vi "数据表比对.vi"(6 "table输入 3":string(combo), 8 "error in (no error)":errorcluster, 9 "查询元素输入":string(combo), 10 "仪器日志参数":string, 11 "table输入":string(combo)) -> (0 "error out":errorcluster, 2 "待发送第一条数据":string[](array[string]), 3 "待发送数据":string[][](table), 4 "获取有效数据":string[][](array[string]))   [LabVIEW 2016]
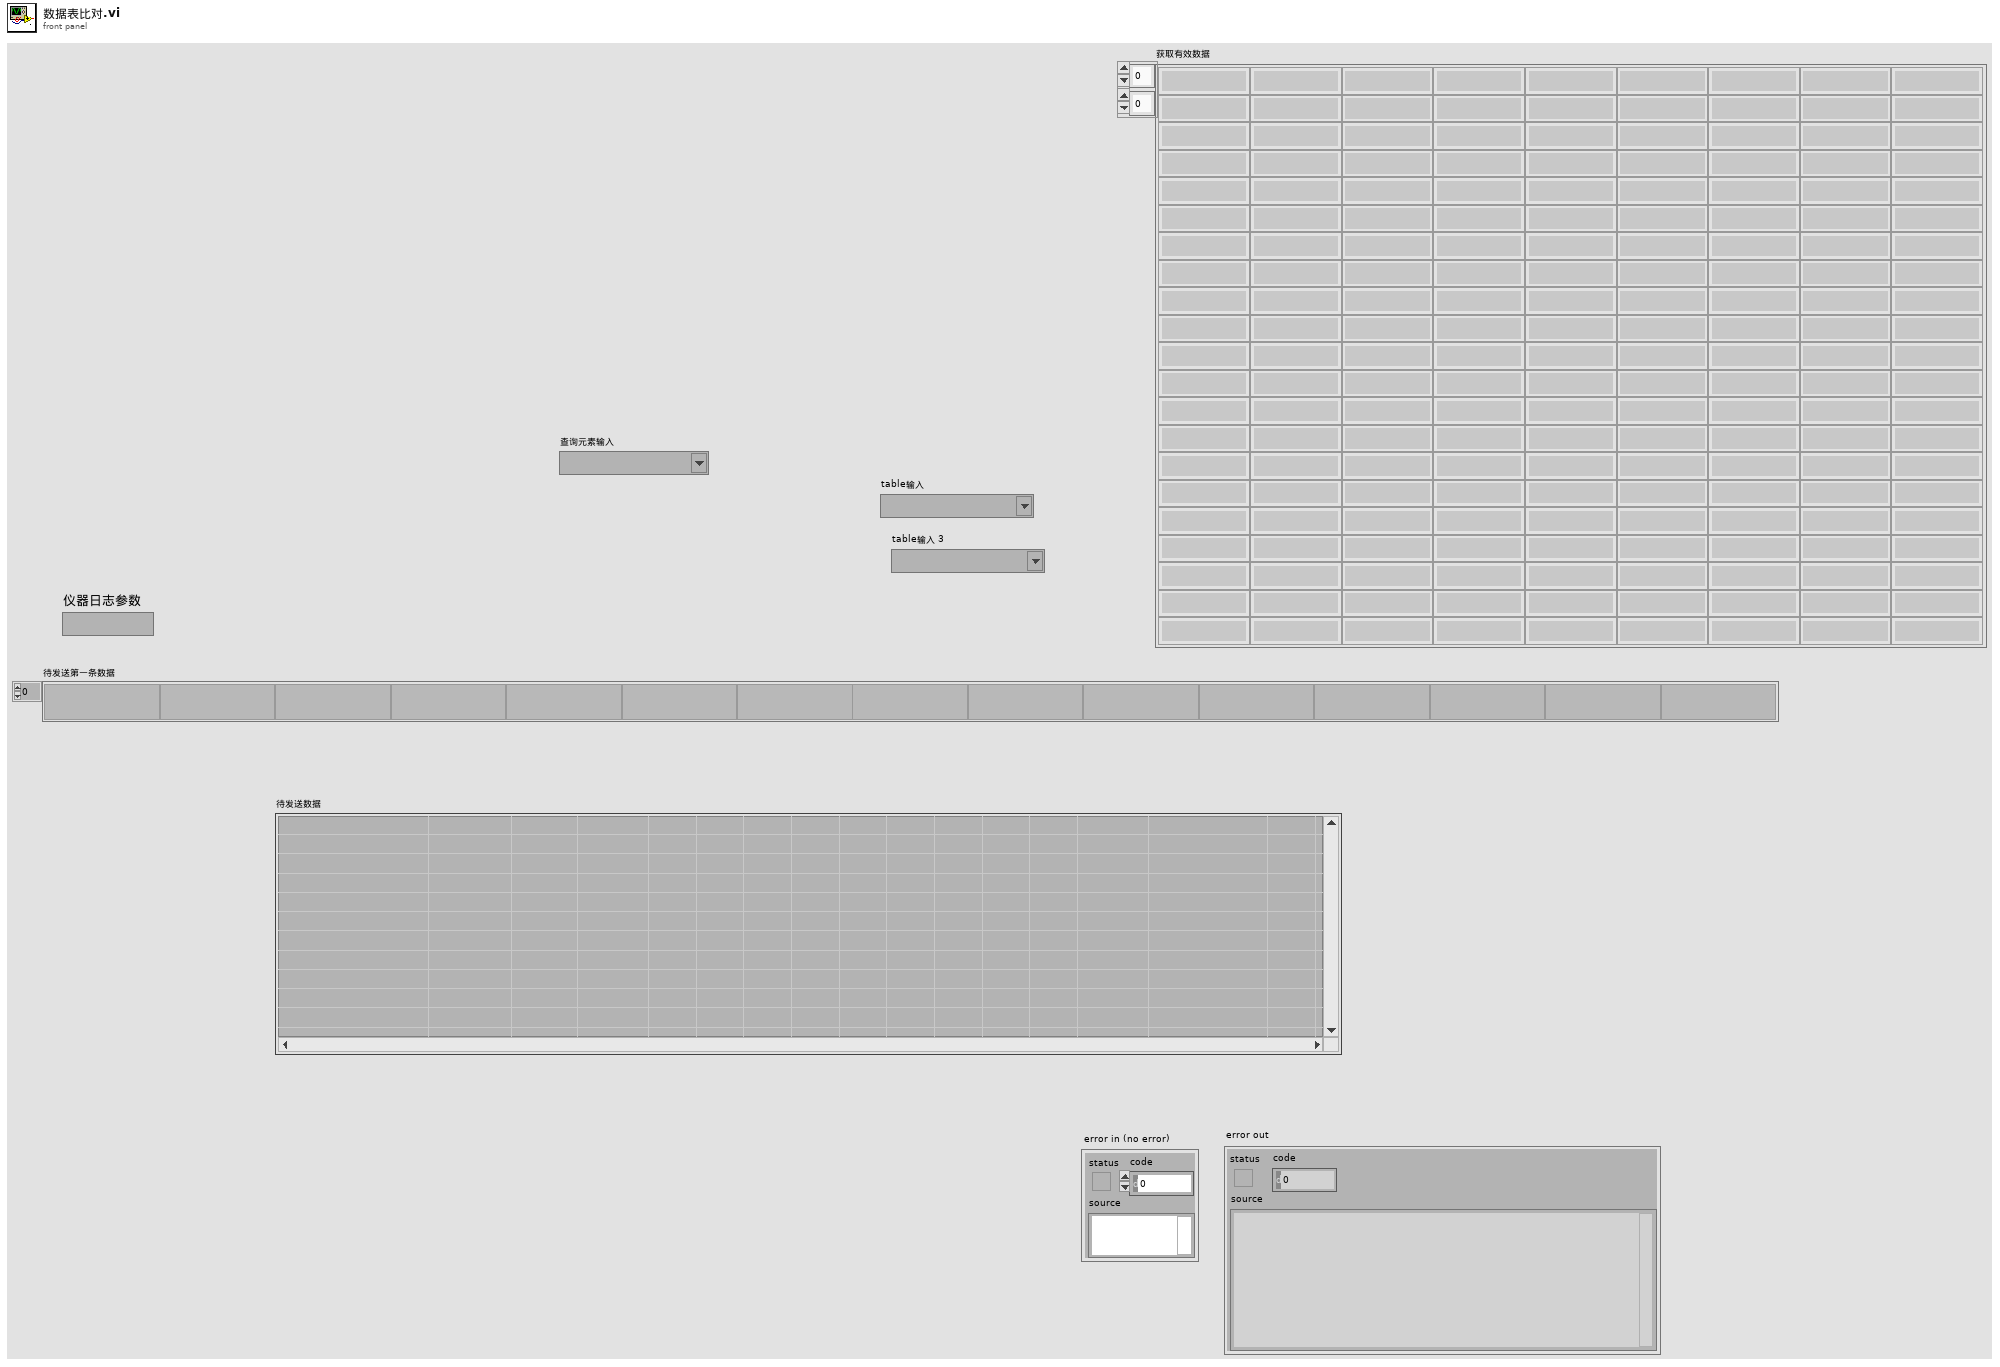
[diagram p1: front panel]
types:
  T1 = typedef "LVDateTimeRec.ctl" = cluster{"秒数的小数部分":dbl, "秒":i32, "分":i32, "时":i32, "日":i32, "月":i32, "年":i32, "天数（周）":i32, "天数（年）":i32, "DST":i32}
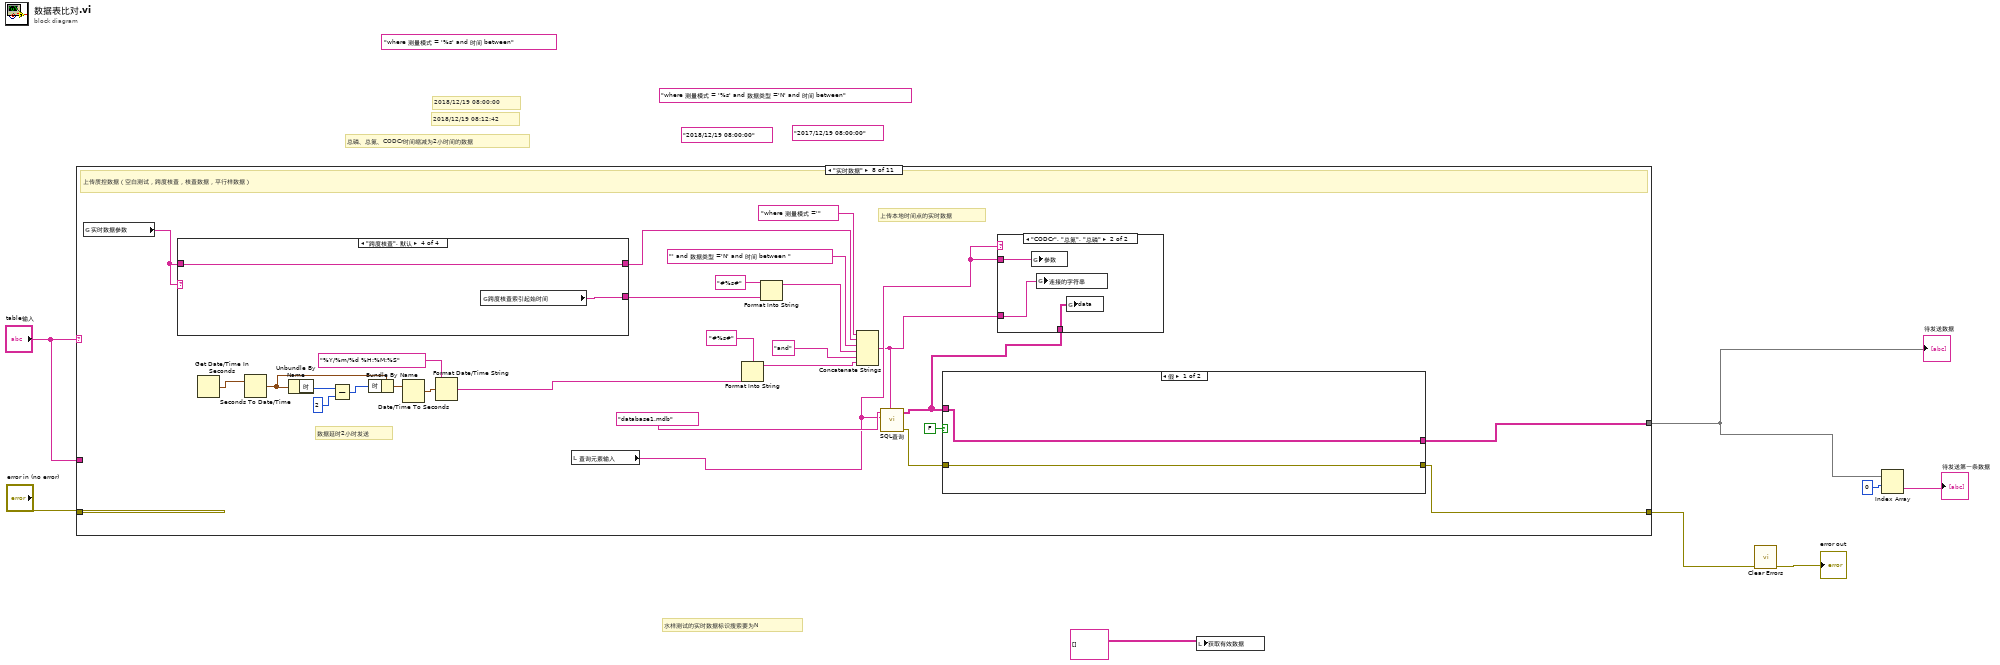
[diagram p0: block diagram]
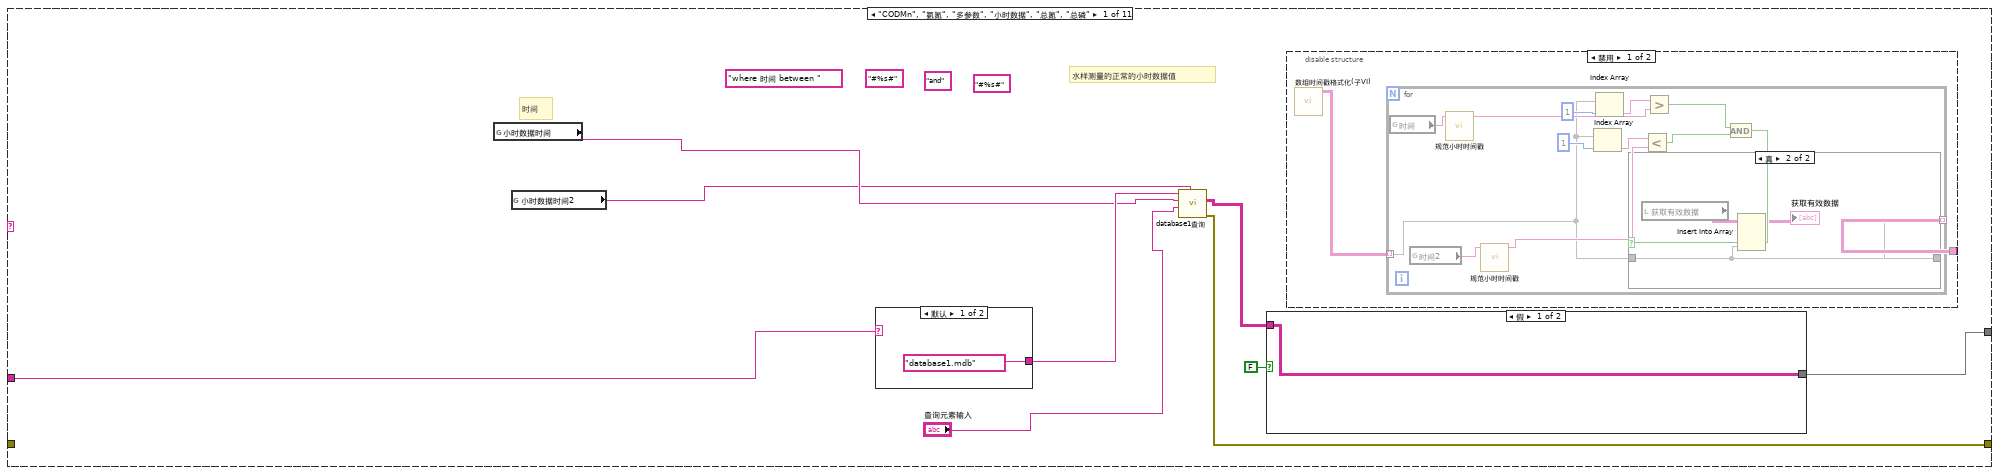
[diagram p2: hidden frame]
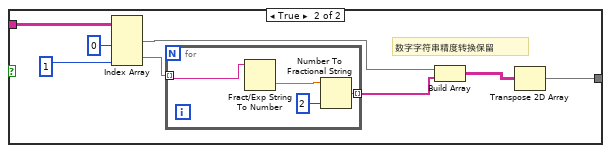
[diagram p3: hidden frame]
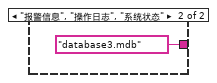
[diagram p6: hidden frame]
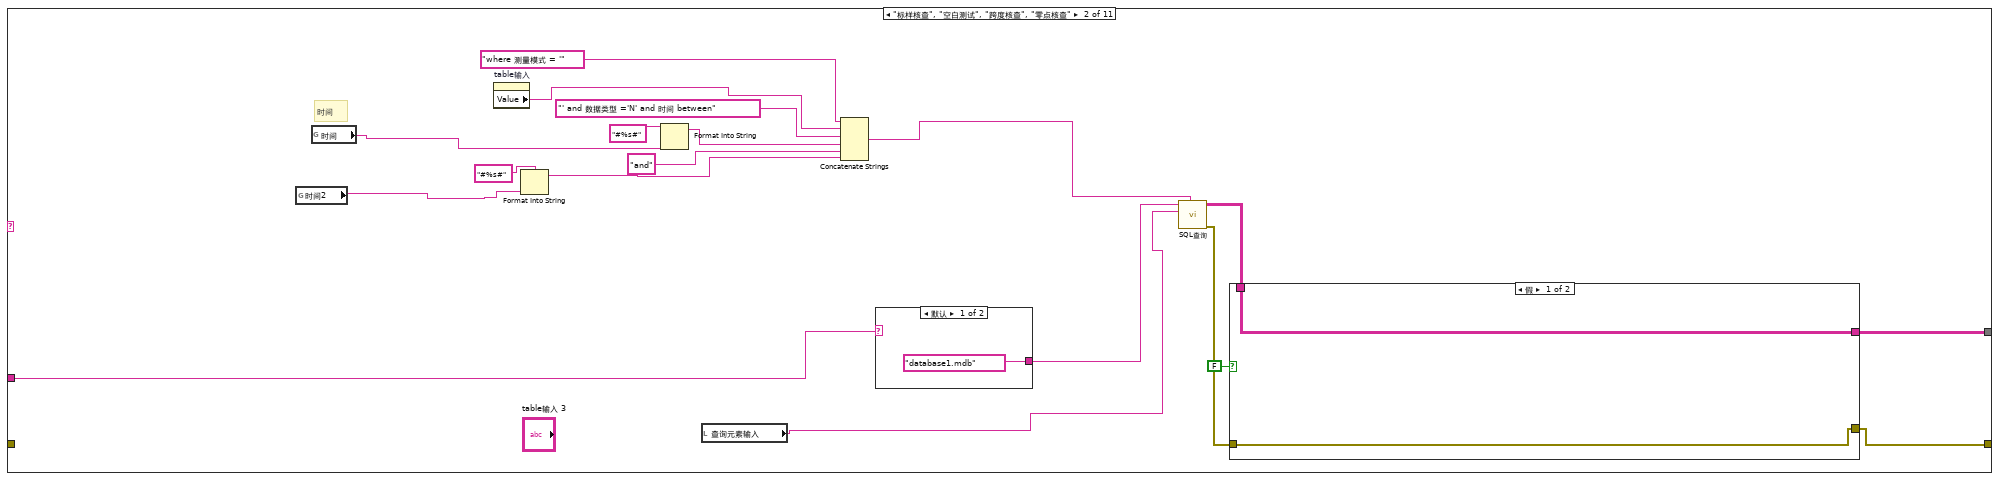
[diagram p7: hidden frame]
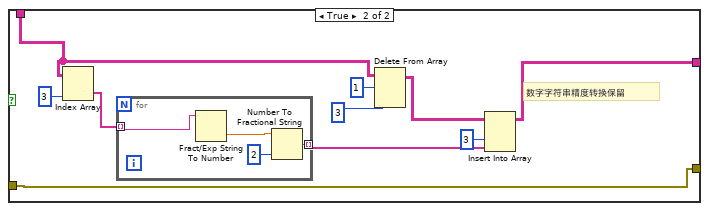
[diagram p8: hidden frame]
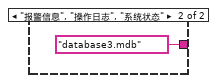
[diagram p9: hidden frame]
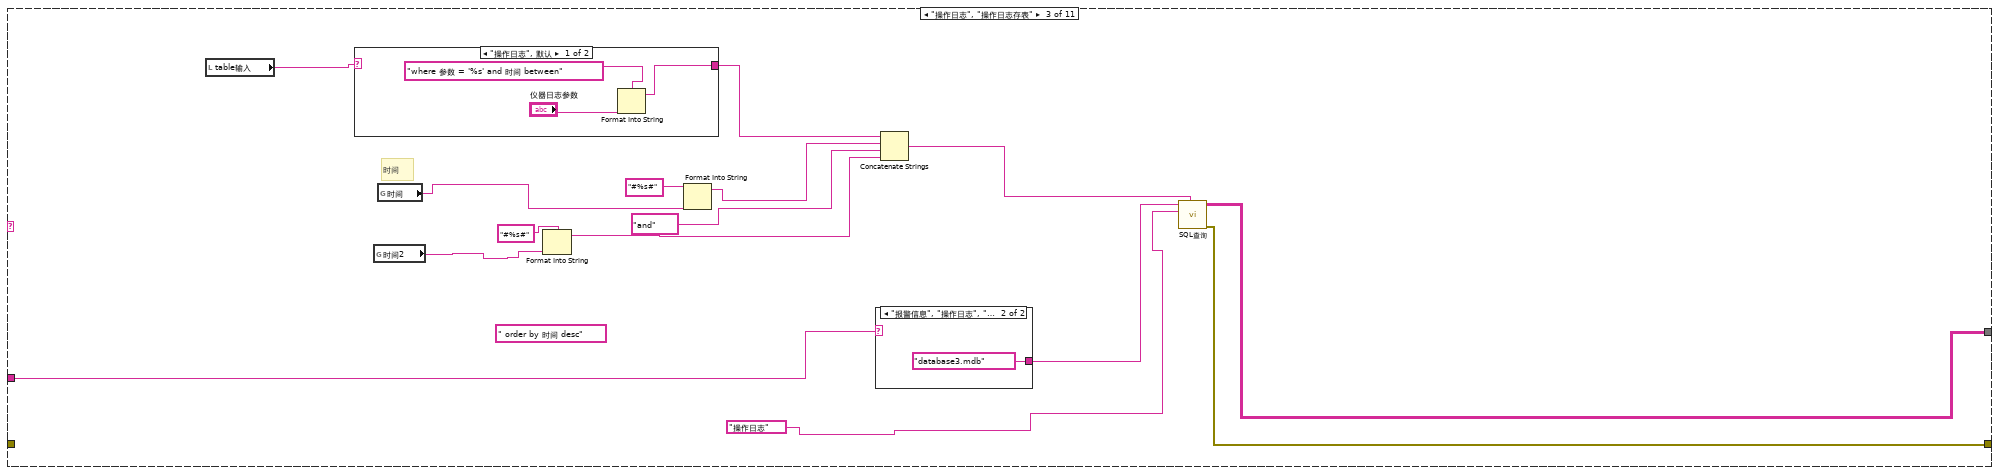
[diagram p10: hidden frame]
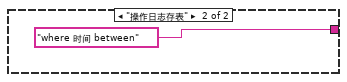
[diagram p11: hidden frame]
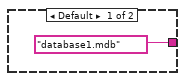
[diagram p12: hidden frame]
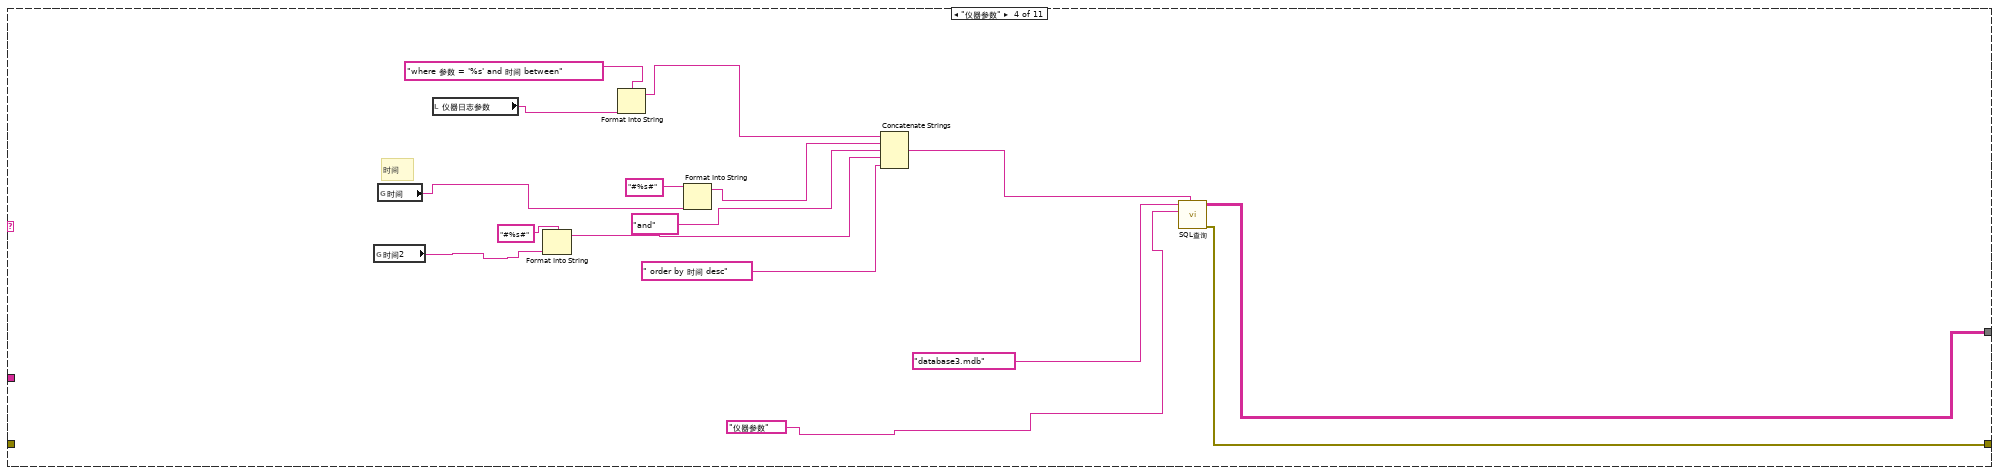
[diagram p13: hidden frame]
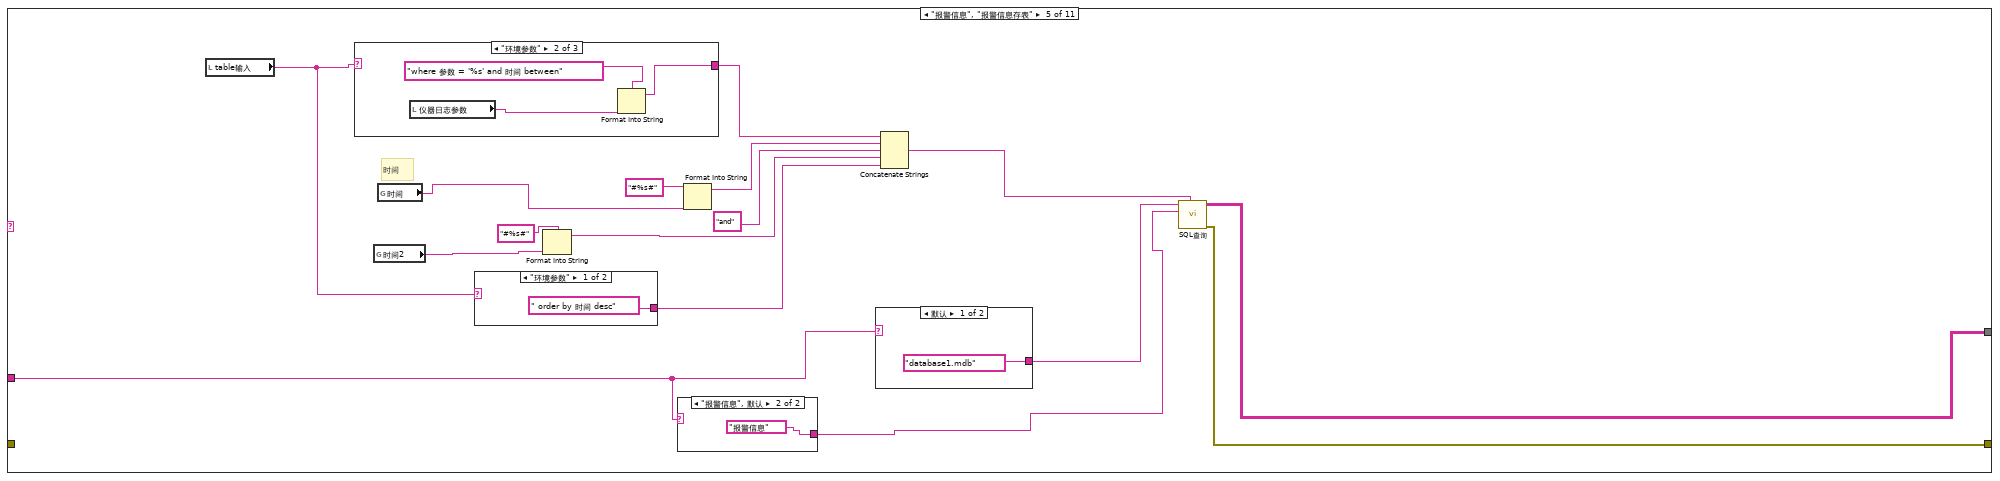
[diagram p14: hidden frame]
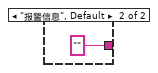
[diagram p15: hidden frame]
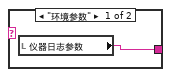
[diagram p16: hidden frame]
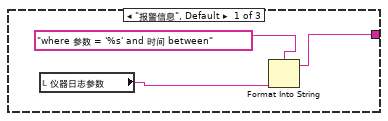
[diagram p17: hidden frame]
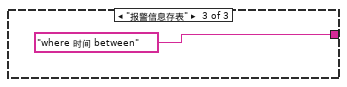
[diagram p18: hidden frame]
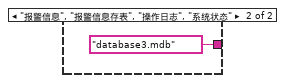
[diagram p19: hidden frame]
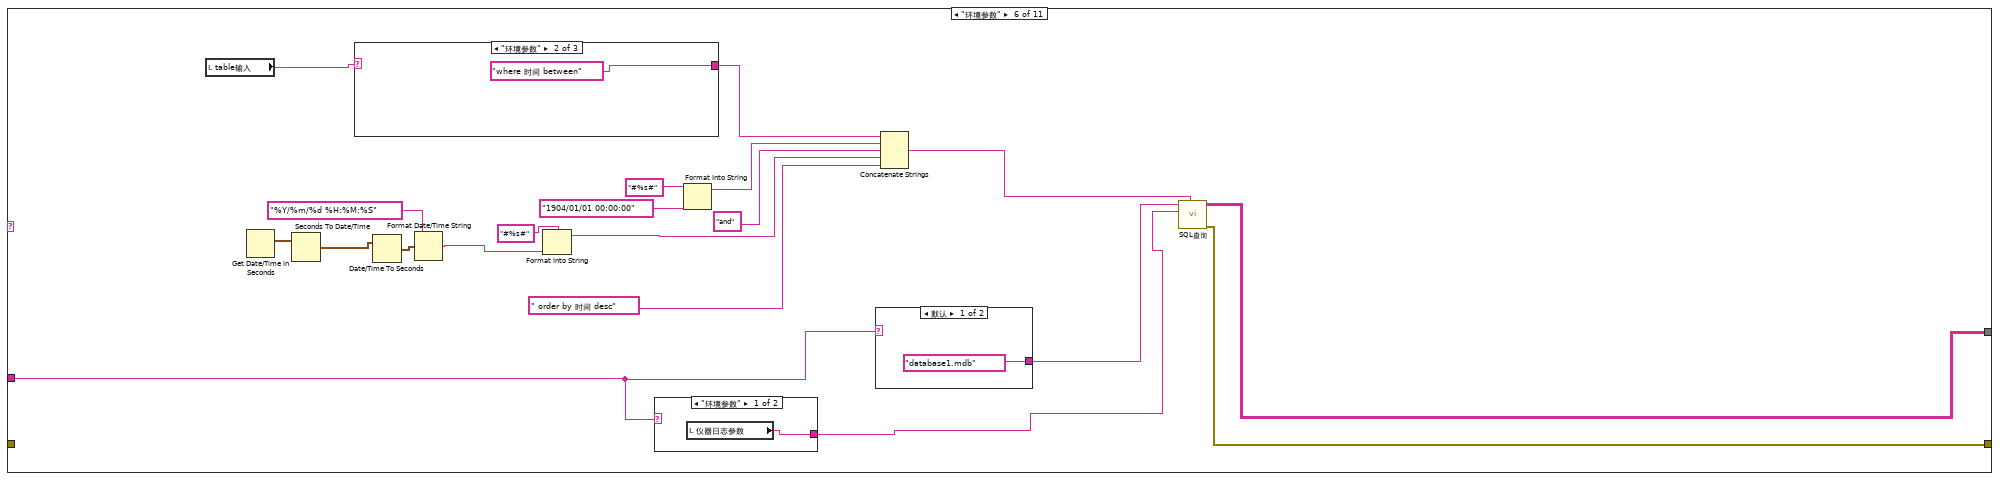
[diagram p20: hidden frame]
diagram:
  (unwired) "where 测量模式 = '%s' and 时间 between" ("condition")
  (unwired) "2017/12/19 08:00:00"
  (unwired) "where 测量模式 = '%s' and 数据类型 ='N' and 时间 between" ("condition")
  (unwired) "2018/12/19 08:00:00"
  # "水样测试的实时数据标识搜索要为N"
  # "2018/12/19 08:00:00"
  # "总磷、总氮、CODCr时间缩减为2小时间的数据"
  # "2018/12/19 08:12:42"
  n1 = case shown="\"实时数据\"" "table输入" {
    tunnel: "error in (no error)" -> [_ _ _ _ _ _ w185 _ _ _ _]
    tunnel: [w14 w55 w100 w123 w139 w172 w185 w201 w266 w309 w349] -> w6
    tunnel: [w10 w58 w98 w121 w137 w170 w183 w204 w269 w312 w351] -> w2
    tunnel: "table输入" -> [w17 w69 w102 _ w127 w162 _ _ _ _ _]
    frame "CODMn", "氨氮", "多参数", "小时数据", "总氮", "总磷" {
      (unwired) "and" ("字符串")
      (unwired) "#%s#" ("初始字符串")
      (unwired) "#%s#" ("初始字符串")
      (unwired) "where 时间 between " ("condition")
      # "水样测量的正常的小时数据值"
      # "时间"
      n2 = global read "全局 水样时间.vi" "小时数据时间"() -> (w13:string)
      n3 = global read "全局 时间2.vi" "小时数据时间2"() -> (w12:string)
      n4 = case shown="默认" w17 {
        tunnel: ["database1.mdb" ("database") "database3.mdb" ("database")] -> w16
        frame Default {
        }
        frame "报警信息", "操作日志", "系统状态" {
        }
      }
      n5 = call "database1查询.vi"("时间2"=w12, "table"="查询元素输入", "时间1"=w13, "database"=w16) -> ("error out"=w14:errorcluster, "data"=w11:string[][])  [unwired: 4 in, 1 out]
      n6 = case shown="假" FALSE {
        tunnel: w11 -> [w18 w26]
        tunnel: [w18 w19] -> w10
        frame False {
        }
        frame True {
          # "数字字符串精度转换保留"
          n7 = Index Array(array=w26, index (col) #1=0 ("禁用的索引 (列)"), index (col) #2=1 ("索引 (列)")) -> (element #1=w22:string[], element #2=w23:string[])  [unwired: 2 in]
          n8 = for {
            tunnel: w23 -> [w28] mode=indexing
            tunnel: [w27] -> w21 mode=indexing
            n9 = Fract/Exp String To Number(string=w28) -> (number=w29:dbl)  [unwired: 3 in, 1 out]
            n10 = Number To Fractional String(number=w29, precision (6)=i16 2 ("精度(6)")) -> (F-format string=w27:string)  [unwired: 2 in]
          }
          n11 = Build Array(w22, w21) -> (w20:string[][])
          n12 = Transpose 2D Array(2D array=w20) -> (transposed array=w19:string[][])
        }
      }
      n13 = disable-structure shown="禁用" {
        disable-tunnel: [w31 _] -> _
        frame Disabled {
          n14 = call "数组时间戳格式化(子VI).vi"() -> ("待发送数据输出"=w32:string[][])  [unwired: 11 in]
          n15 = for {
            tunnel: w32 -> [w33] mode=indexing
            tunnel: [w35] -> w31 mode=indexing
            n16 = global read "全局 水样时间.vi" "时间"() -> (w39:string)
            n17 = global read "全局 时间2.vi" "时间2"() -> (w37:string)
            n18 = call "规范小时时间戳.vi"("字符串"=w39) -> ("result string"=w38:string)  [unwired: 10 in]
            n19 = call "规范小时时间戳.vi"("字符串"=w37) -> ("result string"=w36:string)  [unwired: 10 in]
            n20 = Index Array(array=w33, index=1 ("索引")) -> (element=w42:string)
            n21 = Index Array(array=w33, index=1 ("索引")) -> (element=w44:string)
            n22 = Less?(x=w42, y=w36) -> (x < y?=w41:bool)
            n23 = Greater?(x=w44, y=w38) -> (0:w40:bool)
            n24 = And(x=w40, y=w41) -> (x .and. y?=w34:bool)
            n25 = case shown="真" w34 {
              tunnel: w33 -> [_ w48]
              tunnel: [_ w48] -> w35
              frame False {
              }
              frame True {
                n26 = local read "获取有效数据"() -> (w47:string[][])
                n27 = Insert Into Array(array=w47, new element=w48) -> (→"获取有效数据":string[][])  [unwired: 2 in]
              }
            }
          }
        }
        frame Enabled {
        }
      }
    }
    frame "标样核查", "空白测试", "跨度核查", "零点核查" {
      # "时间"
      n28 = global read "全局 时间2.vi" "时间2"() -> (w60:string)
      n29 = global read "全局 水样时间.vi" "时间"() -> (w61:string)
      n30 = property on="table输入" class="CmbBox"() -> ("Value"=w51:string)  [unwired: 2 in, 2 out]
      n31 = Format Into String(format string="#%s#" ("初始字符串"), w60) -> (resulting string=w63:string)  [unwired: 2 in, 1 out]
      n32 = Format Into String(format string="#%s#" ("初始字符串"), w61) -> (resulting string=w67:string)  [unwired: 2 in, 1 out]
      n33 = local read "查询元素输入"() -> (w54:string)
      n34 = Concatenate Strings("where 测量模式 = '" ("condition"), w51, "' and 数据类型 ='N' and 时间 between" ("字符串"), w67, "and" ("字符串"), w63) -> (w62:string)
      n35 = case shown="默认" w69 {
        tunnel: ["database1.mdb" ("database") "database3.mdb" ("database")] -> w68
        frame Default {
        }
        frame "报警信息", "操作日志", "系统状态" {
        }
      }
      n36 = call "SQL查询.vi"("condition"=w62, "table输入"=w54, "database"=w68) -> ("error out"=w56:errorcluster, "data"=w59:string[][])  [unwired: 7 in]
      n37 = case shown="假" FALSE {
        tunnel: w59 -> [w71 w74]
        tunnel: [w71 w73] -> w58
        tunnel: [w70 w72] -> w55
        tunnel: w56 -> [w70 w72]
        frame False {
        }
        frame True {
          # "数字字符串精度转换保留"
          n38 = Index Array(array=w74, index (col)=3 ("禁用的索引 (列)")) -> (element=w80:string[])  [unwired: 1 in]
          n39 = for {
            tunnel: w80 -> [w83] mode=indexing
            tunnel: [w82] -> w76 mode=indexing
            n40 = Fract/Exp String To Number(string=w83) -> (number=w84:dbl)  [unwired: 3 in, 1 out]
            n41 = Number To Fractional String(number=w84, precision (6)=i16 2 ("精度(6)")) -> (F-format string=w82:string)  [unwired: 2 in]
          }
          n42 = Delete From Array(array=w74, length=1 ("长度"), index (col)=3 ("禁用的索引 (列)")) -> (array with subset deleted=w77:string[][])  [unwired: 1 in, 1 out]
          n43 = Insert Into Array(array=w77, index (col)=3 ("禁用的索引 (列)"), new element=w76) -> (w73:string[][])  [unwired: 1 in]
        }
      }
    }
    frame "操作日志", "操作日志存表" {
      (unwired) " order by 时间 desc" ("字符串")
      # "时间"
      n44 = local read "table输入"() -> (w90:string)
      n45 = case shown="\"操作日志\", 默认" w90 {
        tunnel: [w103 "where 时间 between" ("condition")] -> w89
        frame "操作日志", Default {
          n46 = Format Into String(format string="where 参数 = '%s' and 时间 between" ("condition"), "仪器日志参数") -> (resulting string=w103:string)  [unwired: 2 in, 1 out]
        }
        frame "操作日志存表" {
        }
      }
      n47 = global read "全局 时间2.vi" "时间2"() -> (w91:string)
      n48 = global read "全局 水样时间.vi" "时间"() -> (w92:string)
      n49 = Format Into String(format string="#%s#" ("初始字符串"), w91) -> (resulting string=w93:string)  [unwired: 2 in, 1 out]
      n50 = Format Into String(format string="#%s#" ("初始字符串"), w92) -> (resulting string=w97:string)  [unwired: 2 in, 1 out]
      n51 = case shown="\"报警信息\", \"操作日志\", \"操作日志存表\", \"系统状态\"" w102 {
        tunnel: ["database1.mdb" ("database") "database3.mdb" ("database")] -> w101
        frame Default {
        }
        frame "报警信息", "操作日志", "操作日志存表", "系统状态" {
        }
      }
      n52 = Concatenate Strings(w89, w97, "and" ("字符串"), w93) -> (w99:string)
      n53 = call "SQL查询.vi"("condition"=w99, "table输入"="操作日志", "database"=w101) -> ("error out"=w100:errorcluster, "data"=w98:string[][])  [unwired: 7 in]
    }
    frame "仪器参数" {
      # "时间"
      n54 = global read "全局 时间2.vi" "时间2"() -> (w114:string)
      n55 = global read "全局 水样时间.vi" "时间"() -> (w115:string)
      n56 = local read "仪器日志参数"() -> (w109:string)
      n57 = Format Into String(format string="#%s#" ("初始字符串"), w114) -> (resulting string=w116:string)  [unwired: 2 in, 1 out]
      n58 = Format Into String(format string="where 参数 = '%s' and 时间 between" ("condition"), w109) -> (resulting string=w113:string)  [unwired: 2 in, 1 out]
      n59 = Format Into String(format string="#%s#" ("初始字符串"), w115) -> (resulting string=w120:string)  [unwired: 2 in, 1 out]
      n60 = Concatenate Strings(w113, w120, "and" ("字符串"), w116, " order by 时间 desc" ("字符串")) -> (w122:string)
      n61 = call "SQL查询.vi"("condition"=w122, "table输入"="仪器参数", "database"="database3.mdb") -> ("error out"=w123:errorcluster, "data"=w121:string[][])  [unwired: 7 in]
    }
    frame "报警信息", "报警信息存表" {
      # "时间"
      n62 = local read "table输入"() -> (w126:string)
      n63 = case shown="\"环境参数\"" w126 {
        tunnel: [w146 w149 "where 时间 between" ("condition")] -> w129
        frame "报警信息", Default {
          n64 = local read "仪器日志参数"() -> (w145:string)
          n65 = Format Into String(format string="where 参数 = '%s' and 时间 between" ("condition"), w145) -> (resulting string=w146:string)  [unwired: 2 in, 1 out]
        }
        frame "环境参数" {
          n66 = local read "仪器日志参数"() -> (w148:string)
          n67 = Format Into String(format string="where 参数 = '%s' and 时间 between" ("condition"), w148) -> (resulting string=w149:string)  [unwired: 2 in, 1 out]
        }
        frame "报警信息存表" {
        }
      }
      n68 = global read "全局 时间2.vi" "时间2"() -> (w130:string)
      n69 = global read "全局 水样时间.vi" "时间"() -> (w131:string)
      n70 = case shown="\"环境参数\"" w126 {
        tunnel: [" order by 时间 desc" ("字符串") "" ("仪器日志参数")] -> w125
        frame "环境参数" {
        }
        frame "报警信息", Default {
        }
      }
      n71 = Format Into String(format string="#%s#" ("初始字符串"), w130) -> (resulting string=w132:string)  [unwired: 2 in, 1 out]
      n72 = case shown="\"报警信息\", 默认" w127 {
        tunnel: [w143 "报警信息" ("table输入")] -> w128
        frame "环境参数" {
          n73 = local read "仪器日志参数"() -> (w143:string)
        }
        frame "报警信息", Default {
        }
      }
      n74 = Format Into String(format string="#%s#" ("初始字符串"), w131) -> (resulting string=w136:string)  [unwired: 2 in, 1 out]
      n75 = case shown="默认" w127 {
        tunnel: ["database1.mdb" ("database") "database3.mdb" ("database")] -> w140
        frame Default {
        }
        frame "报警信息", "报警信息存表", "操作日志", "系统状态" {
        }
      }
      n76 = Concatenate Strings(w129, w136, "and" ("字符串"), w132, w125) -> (w138:string)
      n77 = call "SQL查询.vi"("condition"=w138, "table输入"=w128, "database"=w140) -> ("error out"=w139:errorcluster, "data"=w137:string[][])  [unwired: 7 in]
    }
    frame "环境参数" {
      n78 = local read "table输入"() -> (w161:string)
      n79 = Get Date/Time In Seconds() -> (seconds since 1Jan1904=w158:timestamp)
      n80 = Seconds To Date/Time(time stamp (now)=w158) -> (date time rec=w155:T1)  [unwired: 1 in]
      n81 = case shown="\"环境参数\"" w161 {
        tunnel: [w177 "where 时间 between" ("condition") "where 时间 between" ("condition")] -> w164
        frame "报警信息", Default {
          n82 = local read "仪器日志参数"() -> (w176:string)
          n83 = Format Into String(format string="where 参数 = '%s' and 时间 between" ("condition"), w176) -> (resulting string=w177:string)  [unwired: 2 in, 1 out]
        }
        frame "环境参数" {
        }
        frame "报警信息存表" {
        }
      }
      n84 = Date/Time To Seconds(2:w155) -> (0:w157:timestamp)  [unwired: 1 in]
      n85 = Format Date/Time String(time format string (%c)="%Y/%m/%d %H:%M:%S" ("时间格式字符串(%c)"), seconds (now)=w157) -> (date/time string=w154:string)  [unwired: 1 in]
      n86 = Format Into String(format string="#%s#" ("初始字符串"), w154) -> (resulting string=w165:string)  [unwired: 2 in, 1 out]
      n87 = case shown="\"环境参数\"" w162 {
        tunnel: [w174 "报警信息" ("table输入")] -> w163
        frame "环境参数" {
          n88 = local read "仪器日志参数"() -> (w174:string)
        }
        frame "报警信息", Default {
        }
      }
      n89 = Format Into String(format string="#%s#" ("初始字符串"), "1904/01/01 00:00:00") -> (resulting string=w169:string)  [unwired: 2 in, 1 out]
      n90 = case shown="默认" w162 {
        tunnel: ["database1.mdb" ("database") "database3.mdb" ("database")] -> w173
        frame Default {
        }
        frame "报警信息", "报警信息存表", "操作日志", "系统状态" {
        }
      }
      n91 = Concatenate Strings(w164, w169, "and" ("字符串"), w165, " order by 时间 desc" ("字符串")) -> (w171:string)
      n92 = call "SQL查询.vi"("condition"=w171, "table输入"=w163, "database"=w173) -> ("error out"=w172:errorcluster, "data"=w170:string[][])  [unwired: 7 in]
    }
    frame Default {
      # "时间格式转换"
      n93 = local read "待发送数据"() -> (w184:string[][])
      n94 = call "数组时间戳格式化(子VI).vi"("待发送数据输入"=w184) -> ("待发送数据输出"=w183:string[][])  [unwired: 10 in]
    }
    frame "实时数据" {
      # "数据延时2小时发送"
      # "上传本地时间点的实时数据"
      # "上传质控数据（空白测试，跨度核查，核查数据，平行样数据）"
      n95 = global read "全局 实时数据参数.vi" "实时数据参数"() -> (w196:string)
      n96 = case shown="\"跨度核查\", 默认" w196 {
        tunnel: [w214 w231 w233 w235] -> w197
        tunnel: w196 -> [w213 w230 _ w234]
        tunnel: [w213 w230 "标样核查" ("实时数据参数") w234] -> w195
        frame "水样测试" {
          n97 = Get Date/Time In Seconds() -> (seconds since 1Jan1904=w222:timestamp)
          n98 = local read "查询元素输入"() -> (w215:string)
          n99 = Format Date/Time String(time format string (%c)="%Y%m%d%H%M%S%3u" ("时间格式字符串(%c)"), seconds (now)=w222) -> (date/time string=w220:string)  [unwired: 1 in]
          n100 = Replace Substring(2:8 ("长度（子字符串长度）"), 3:10 ("偏移量(0)"), 4:"0000" ("子字符串(\"\")"), 5:w220) -> (1:w216:string)  [unwired: 1 out]
          n101 = case shown="默认" w215 {
            tunnel: w216 -> [w224 w227 _]
            tunnel: [w223 w228 w229] -> w214
            frame Default {
              n102 = Search and Replace String(input string=w224, search string="." ("搜索字符串")) -> (result string=w225:string)  [unwired: 6 in, 3 out]
              n103 = call "格式时间字符串.vi"("字符串"=w225) -> ("连接的字符串"=w223:string)  [unwired: 10 in]
            }
            frame "CODCr", "CODMn", "累积流量", "总氮", "总磷" {
              n104 = call "实时数据查询用2小时间的数据.vi"("字符串"=w227) -> ("连接的字符串"=w228:string)  [unwired: 10 in]
            }
            frame "CODCr加标回收率", "CODMn加标回收率", "氨氮加标回收率", "总氮加标回收率", "总磷加标回收率" {
              n105 = global read "全局 时间2.vi" "加标回收索引起始时间"() -> (w229:string)
            }
          }
        }
        frame "空白测试" {
          n106 = global read "全局 时间2.vi" "零点核查索引起始时间"() -> (w231:string)
        }
        frame "核查数据" {
          n107 = global read "全局 时间2.vi" "标样核查索引起始时间"() -> (w233:string)
        }
        frame "跨度核查", Default {
          n108 = global read "全局 时间2.vi" "跨度核查索引起始时间"() -> (w235:string)
        }
      }
      n109 = Get Date/Time In Seconds() -> (seconds since 1Jan1904=w194:timestamp)
      n110 = Seconds To Date/Time(time stamp (now)=w194) -> (date time rec=w193:T1)  [unwired: 1 in]
      n111 = Unbundle By Name(w193) -> ("时"=w189:i32)
      n112 = Subtract(x=w189, y=2) -> (x-y=w188:i32)
      n113 = Bundle By Name(cluster=w193, "时"=w188) -> (w191:T1)
      n114 = Date/Time To Seconds(2:w191) -> (0:w192:timestamp)  [unwired: 1 in]
      n115 = Format Date/Time String(time format string (%c)="%Y/%m/%d %H:%M:%S" ("时间格式字符串(%c)"), seconds (now)=w192) -> (date/time string=w186:string)  [unwired: 1 in]
      n116 = local read "查询元素输入"() -> (w200:string)
      n117 = Format Into String(format string="#%s#" ("初始字符串"), w186) -> (resulting string=w208:string)  [unwired: 2 in, 1 out]
      n118 = Format Into String(format string="#%s#" ("初始字符串"), w197) -> (resulting string=w212:string)  [unwired: 2 in, 1 out]
      n119 = Concatenate Strings("where 测量模式 ='" ("condition"), w195, "' and 数据类型 ='N' and 时间 between ", w212, "and" ("字符串"), w208) -> (w199:string)
      n120 = call "SQL查询.vi"("condition"=w199, "table输入"=w200, "database"="database1.mdb") -> ("error out"=w202:errorcluster, "data"=w198:string[][])  [unwired: 7 in]
      n121 = case shown="假" FALSE {
        tunnel: [w240 w243] -> w204
        tunnel: w198 -> [w240 w242]
        tunnel: w202 -> [w239 w241]
        tunnel: [w239 w241] -> w201
        frame False {
        }
        frame True {
          # "数字字符串精度转换保留"
          n122 = Index Array(array=w242, index (col)=3 ("禁用的索引 (列)")) -> (element=w249:string[])  [unwired: 1 in]
          n123 = for {
            tunnel: w249 -> [w252] mode=indexing
            tunnel: [w251] -> w245 mode=indexing
            n124 = Fract/Exp String To Number(string=w252) -> (number=w253:dbl)  [unwired: 3 in, 1 out]
            n125 = Number To Fractional String(number=w253, precision (6)=i16 2 ("精度(6)")) -> (F-format string=w251:string)  [unwired: 2 in]
          }
          n126 = Delete From Array(array=w242, length=1 ("长度"), index (col)=3 ("禁用的索引 (列)")) -> (array with subset deleted=w246:string[][])  [unwired: 1 in, 1 out]
          n127 = Insert Into Array(array=w246, index (col)=3 ("禁用的索引 (列)"), new element=w245) -> (w243:string[][])  [unwired: 1 in]
        }
      }
      n128 = case shown="\"CODCr\", \"总氮\", \"总磷\"" w200 {
        tunnel: w200 -> [_ w238]
        tunnel: w199 -> [_ w237]
        tunnel: w198 -> [_ w236]
        frame Default {
        }
        frame "CODCr", "总氮", "总磷" {
          n129 = global write "全局 实时数据参数.vi" "参数"(w238) -> ()
          n130 = global write "全局 实时数据参数.vi" "连接的字符串"(w237) -> ()
          n131 = global write "全局 实时数据参数.vi" "data"(w236) -> ()
        }
      }
    }
    frame "加标回收" {
      w261 = "加标回收率" ("字符串")
      # "上传本地时间点的实时数据"
      # "上传加标回收数据"
      n132 = global read "全局 数据发送重叠.vi" "掉线指示灯"() -> (w262:bool)
      n133 = case shown="假" w262 {
        tunnel: [w278 w282] -> w263
        frame False {
          n134 = global read "全局 数据发送重叠.vi" "数据发送重叠"() -> (w279:bool)
          n135 = case shown="假" w279 {
            tunnel: [w280 w281] -> w278
            frame False {
              n136 = global read "全局 时间2.vi" "加标回收索引起始时间"() -> (w280:string)
            }
            frame True {
              n137 = global read "全局 数据发送重叠.vi" "数据发送重叠开始时间戳"() -> (w281:string)
            }
          }
        }
        frame True {
          n138 = global read "全局 数据发送重叠.vi" "TCP掉线时间节点"() -> (w282:string)
        }
      }
      n139 = Get Date/Time In Seconds() -> (seconds since 1Jan1904=w259:timestamp)
      n140 = Seconds To Date/Time(time stamp (now)=w259) -> (date time rec=w256:T1)  [unwired: 1 in]
      n141 = Date/Time To Seconds(2:w256) -> (0:w258:timestamp)  [unwired: 1 in]
      n142 = Format Date/Time String(time format string (%c)="%Y/%m/%d %H:%M:%S" ("时间格式字符串(%c)"), seconds (now)=w258) -> (date/time string=w255:string)  [unwired: 1 in]
      n143 = local read "查询元素输入"() -> (w260:string)
      n144 = Format Into String(format string="#%s#" ("初始字符串"), w255) -> (resulting string=w273:string)  [unwired: 2 in, 1 out]
      n145 = Format Into String(format string="#%s#" ("初始字符串"), w263) -> (resulting string=w277:string)  [unwired: 2 in, 1 out]
      n146 = Concatenate Strings("where 参数 ='" ("condition"), w260, "' and 时间 between ", w277, "and" ("字符串"), w273) -> (w265:string)
      n147 = call "SQL查询.vi"("condition"=w265, "table输入"=w261, "database"="database1.mdb") -> ("error out"=w267:errorcluster, "data"=w264:string[][])  [unwired: 7 in]
      n148 = case shown="假" FALSE {
        tunnel: [w287 w290] -> w269
        tunnel: w264 -> [w287 w289]
        tunnel: w267 -> [w286 w288]
        tunnel: [w286 w288] -> w266
        frame False {
        }
        frame True {
          # "数字字符串精度转换保留"
          n149 = Index Array(array=w289, index (col)=3 ("禁用的索引 (列)")) -> (element=w296:string[])  [unwired: 1 in]
          n150 = for {
            tunnel: w296 -> [w299] mode=indexing
            tunnel: [w298] -> w292 mode=indexing
            n151 = Fract/Exp String To Number(string=w299) -> (number=w300:dbl)  [unwired: 3 in, 1 out]
            n152 = Number To Fractional String(number=w300, precision (6)=i16 2 ("精度(6)")) -> (F-format string=w298:string)  [unwired: 2 in]
          }
          n153 = Delete From Array(array=w289, length=1 ("长度"), index (col)=3 ("禁用的索引 (列)")) -> (array with subset deleted=w293:string[][])  [unwired: 1 in, 1 out]
          n154 = Insert Into Array(array=w293, index (col)=3 ("禁用的索引 (列)"), new element=w292) -> (w290:string[][])  [unwired: 1 in]
        }
      }
      n155 = case shown="\"CODCr\", \"总氮\", \"总磷\"" w261 {
        tunnel: w261 -> [_ w285]
        tunnel: w265 -> [_ w284]
        tunnel: w264 -> [_ w283]
        frame Default {
        }
        frame "CODCr", "总氮", "总磷" {
          n156 = global write "全局 实时数据参数.vi" "参数"(w285) -> ()
          n157 = global write "全局 实时数据参数.vi" "连接的字符串"(w284) -> ()
          n158 = global write "全局 实时数据参数.vi" "data"(w283) -> ()
        }
      }
    }
    frame "提取加标回收" {
      w304 = "加标回收率" ("字符串")
      # "上传本地时间点的实时数据"
      n159 = global read "全局 数据发送重叠.vi" "掉线指示灯"() -> (w305:bool)
      n160 = case shown="假" w305 {
        tunnel: [w321 w325] -> w306
        frame False {
          n161 = global read "全局 数据发送重叠.vi" "数据发送重叠"() -> (w322:bool)
          n162 = case shown="假" w322 {
            tunnel: [w323 w324] -> w321
            frame False {
              n163 = global read "起始时间.vi" "起始时间"() -> (w323:string)
            }
            frame True {
              n164 = global read "全局 数据发送重叠.vi" "数据发送重叠开始时间戳"() -> (w324:string)
            }
          }
        }
        frame True {
          n165 = global read "全局 数据发送重叠.vi" "TCP掉线时间节点"() -> (w325:string)
        }
      }
      n166 = global read "起始时间.vi" "结束时间"() -> (w302:string)
      n167 = local read "查询元素输入"() -> (w303:string)
      n168 = Format Into String(format string="#%s#" ("初始字符串"), w302) -> (resulting string=w316:string)  [unwired: 2 in, 1 out]
      n169 = Format Into String(format string="#%s#" ("初始字符串"), w306) -> (resulting string=w320:string)  [unwired: 2 in, 1 out]
      n170 = Concatenate Strings("where 参数 ='" ("condition"), w303, "' and 时间 between ", w320, "and" ("字符串"), w316) -> (w308:string)
      n171 = call "SQL查询.vi"("condition"=w308, "table输入"=w304, "database"="database1.mdb") -> ("error out"=w310:errorcluster, "data"=w307:string[][])  [unwired: 7 in]
      n172 = case shown="假" FALSE {
        tunnel: [w330 w333] -> w312
        tunnel: w307 -> [w330 w332]
        tunnel: w310 -> [w329 w331]
        tunnel: [w329 w331] -> w309
        frame False {
        }
        frame True {
          # "数字字符串精度转换保留"
          n173 = Index Array(array=w332, index (col)=3 ("禁用的索引 (列)")) -> (element=w339:string[])  [unwired: 1 in]
          n174 = for {
            tunnel: w339 -> [w342] mode=indexing
            tunnel: [w341] -> w335 mode=indexing
            n175 = Fract/Exp String To Number(string=w342) -> (number=w343:dbl)  [unwired: 3 in, 1 out]
            n176 = Number To Fractional String(number=w343, precision (6)=i16 2 ("精度(6)")) -> (F-format string=w341:string)  [unwired: 2 in]
          }
          n177 = Delete From Array(array=w332, length=1 ("长度"), index (col)=3 ("禁用的索引 (列)")) -> (array with subset deleted=w336:string[][])  [unwired: 1 in, 1 out]
          n178 = Insert Into Array(array=w336, index (col)=3 ("禁用的索引 (列)"), new element=w335) -> (w333:string[][])  [unwired: 1 in]
        }
      }
      n179 = case shown="\"CODCr\", \"总氮\", \"总磷\"" w304 {
        tunnel: w304 -> [_ w328]
        tunnel: w308 -> [_ w327]
        tunnel: w307 -> [_ w326]
        frame Default {
        }
        frame "CODCr", "总氮", "总磷" {
          n180 = global write "全局 实时数据参数.vi" "参数"(w328) -> ()
          n181 = global write "全局 实时数据参数.vi" "连接的字符串"(w327) -> ()
          n182 = global write "全局 实时数据参数.vi" "data"(w326) -> ()
        }
      }
    }
    frame "提取实时数据" {
      # "上传给定时间段之间的实时数据"
      n183 = global read "起始时间.vi" "起始时间"() -> (w354:string)
      n184 = global read "起始时间.vi" "结束时间"() -> (w353:string)
      n185 = local read "查询元素输入"() -> (w358:string)
      n186 = global read "全局 实时数据参数.vi" "实时数据参数"() -> (w346:string)
      n187 = Format Into String(format string="#%s#" ("初始字符串"), w354) -> (resulting string=w362:string)  [unwired: 2 in, 1 out]
      n188 = Format Into String(format string="#%s#" ("初始字符串"), w353) -> (resulting string=w355:string)  [unwired: 2 in, 1 out]
      n189 = Concatenate Strings("where 测量模式 ='" ("condition"), w346, "' and 时间 between ", w362, "and" ("字符串"), w355) -> (w360:string)
      n190 = call "SQL查询.vi"("condition"=w360, "table输入"=w358, "database"="database1.mdb") -> ("error out"=w350:errorcluster, "data"=w352:string[][])  [unwired: 7 in]
      n191 = case shown="假" FALSE {
        tunnel: w352 -> [w364 w372]
        tunnel: [w364 w366] -> w351
        tunnel: w350 -> [w363 w365]
        tunnel: [w363 w365] -> w349
        frame False {
        }
        frame True {
          # "数字字符串精度转换保留"
          n192 = Index Array(array=w372, index (col)=3 ("禁用的索引 (列)")) -> (element=w373:string[])  [unwired: 1 in]
          n193 = for {
            tunnel: w373 -> [w376] mode=indexing
            tunnel: [w375] -> w368 mode=indexing
            n194 = Fract/Exp String To Number(string=w376) -> (number=w377:dbl)  [unwired: 3 in, 1 out]
            n195 = Number To Fractional String(number=w377, precision (6)=i16 2 ("精度(6)")) -> (F-format string=w375:string)  [unwired: 2 in]
          }
          n196 = Delete From Array(array=w372, length=1 ("长度"), index (col)=3 ("禁用的索引 (列)")) -> (array with subset deleted=w369:string[][])  [unwired: 1 in, 1 out]
          n197 = Insert Into Array(array=w369, index (col)=3 ("禁用的索引 (列)"), new element=w368) -> (w366:string[][])  [unwired: 1 in]
        }
      }
    }
  }
  "待发送数据" <- w2
  n198 = local write "获取有效数据"(string[][] []) -> ()
  n199 = call <vilib>:"Clear Errors.vi"("error in (no error)"=w6) -> ("error out"=→"error out":errorcluster)  [unwired: 5 in, 1 out]
  n200 = Index Array(array=w2, index (row)=0 ("索引 (行)")) -> (element=→"待发送第一条数据":string[])  [unwired: 1 in]
